vi "Actor Destroy Decorator.vi"(11 "Dev Actor in":refnum<class "Dev Actor.lvclass">) -> (0 "error out":errorcluster, 3 "Dev Actor out":refnum<class "Dev Actor.lvclass">)   [LabVIEW 2021, in "Dev Actor.lvlib" / "Dev Actor.lvclass"]
uses:
  Dev Actor.lvclass
  Dev Actor.lvclass/Dev Actor.ctl
  src/LVCAM/LVCAM/Actor/Actor.lvclass
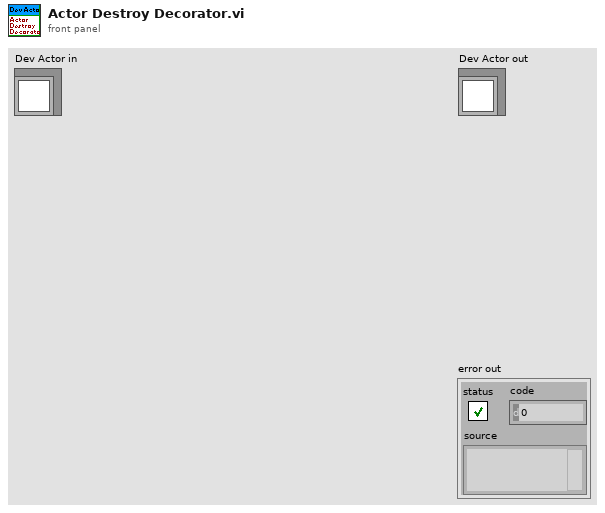
[diagram p1: front panel]
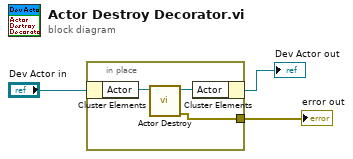
[diagram p0: block diagram]
diagram:
  n1 = in-place {
    in-place-border: [w4] -> w1
    n2 = in-place-cluster #1("Dev Actor in") -> ("Actor"=w6:refnum<class "Actor.lvclass">)
    n3 = call-dynamic "Actor Destroy.vi"("Actor Destroy in"=w6) -> ("error out"=w4:errorcluster, "Actor Destroy out"=w5:refnum<class "Actor.lvclass">)  [unwired: 9 in]
    n4 = in-place-cluster #1("Actor"=w5) -> (→"Dev Actor out":refnum<class "Dev Actor.lvclass">)
  }
  "error out" <- w1
